vi "SeCrTs-Continuous or cummulative DI.vi"(8 "DI   data":bool[](array[boolean]), 9 "DI Channels Name":string[](array[string]), 10 "CDT":dbl, 11 "output cluster":T1) -> (2 "Failure case Seq":string, 3 "In Range":string)   [LabVIEW 2022 SP3]
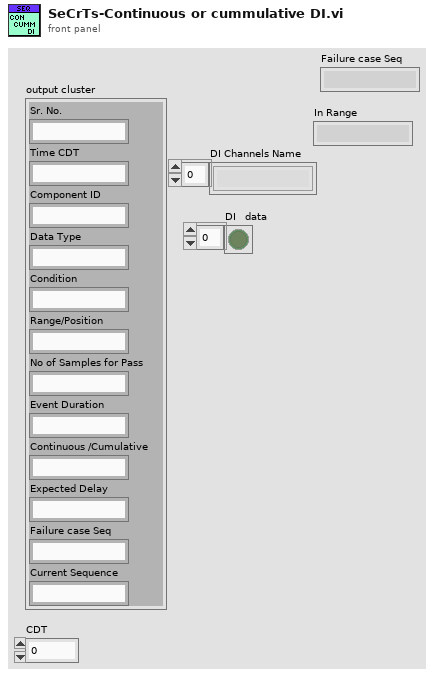
[diagram p1: front panel]
types:
  T1 = cluster{"Sr. No.":string, "Time CDT":string, "Component ID":string, "Data Type":string, "Condition":string, "Range/Position":string, "No of Samples for Pass":string, "Event Duration":string, "Continuous /Cumulative":string, "Expected Delay":string, "Failure case Seq":string, "Current Sequence":string}
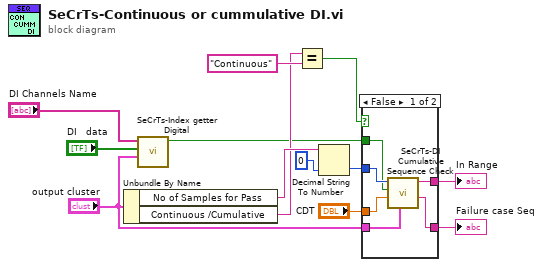
[diagram p0: block diagram]
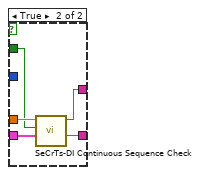
[diagram p2: hidden frame]
diagram:
  n1 = Unbundle By Name("output cluster") -> ("No of Samples for Pass"=w10:string, "Continuous /Cumulative"=w6:string)
  n2 = call "SeCrTs-Index getter  Digital.vi"("output cluster"="output cluster", "DI Y  data"="DI   data", "DI Channels Name"="DI Channels Name") -> ("Digital data"=w5:bool)  [unwired: 8 in]
  n3 = Equal?(x=w6, y="Continuous") -> (x = y?=w8:bool)
  n4 = Decimal String To Number(string=w10, default (0L)=0) -> (number=w11:i32)  [unwired: 1 in, 1 out]
  n5 = case shown="False" w8 {
    tunnel: w5 -> [w15 w21]
    tunnel: "output cluster" -> [w17 w23]
    tunnel: w11 -> [w19 _]
    tunnel: [w16 w22] -> w4
    tunnel: "CDT" -> [w18 w24]
    tunnel: [w14 w20] -> w1
    frame False {
      n6 = call "SeCrTs-DI Cumulative Sequence Check.vi"("output cluster"=w17, "CDT"=w18, "DI Data"=w15, "Numeric 2"=w19) -> ("Failure case Seq"=w14:string, "String"=w16:string)  [unwired: 5 in, 1 out]
    }
    frame True {
      n7 = call "SeCrTs-DI Continuous Sequence Check.vi"("output cluster"=w23, "DI"=w21, "CDT"=w24) -> ("Failure case Seq"=w20:string, "In Range"=w22:string)  [unwired: 6 in, 1 out]
    }
  }
  "In Range" <- w4
  "Failure case Seq" <- w1
